vi "Detector Init.vi"(8 "error in (no error)":errorcluster, 10 "Detector Config":T2={"Detector"=0, "Offsets"=[[0, 0, 0, 0, 0, 0, 0, 0, 0, 0, 0, 0, 0, 0, 0, 0, 0, 0, 0, 0, 0, 0, 0, 0, 0, 0, 0, 0, 0, 0, 0, 0]], "Detector Computer"={"Machine"="192.168.121.11", "Password"="", "FITS File Path"="", "Port"=44444, "Header Path"="", "Name"=""}, "FITS hdr template0"=path "", "FITS hdr template1"=path "", "FITS Data File Path"=path "", "FITS Detector Settings"={"Exp Time Short"=0.0, "# of Frames"=0.0, "Exp Time Long"=0.0, "# of Groups"=0.0, "Object Name"="", "Object"="", "Obs Type"="", "Image Type"="", "Observer"="", "Observer Affiliation"=""}, "Sim Folder"=path "", "Integration Mode"=enum."Ramp", "Integration Time"=0.0, "Frame Int Time"=0.0} {"Offsets" format="%04x"; "Detector" items=["0", "1", "2"]}, 11 "PRIME Detector in":refnum<class "PRIME Detector.lvclass">) -> (0 "error out":errorcluster, 2 "Log Messages":string[](array[string]), 3 "PRIME Detector out":refnum<class "PRIME Detector.lvclass">)   [LabVIEW 2024, in "PRIME Detector.lvclass"]
uses:
  PRIME Detector.lvclass
  RIMAS Detector Config.ctl
  RIMAS Detector Server Config.ctl
  RIMAS Observation Config.ctl
  Detector enum Detector Integration Mode.ctl
  PRIME Detector cluster Status.ctl
  PRIME Detector.lvclass/PRIME Detector.ctl
  Detector Class.lvclass
panel:
  out "Status":T1
  # "sec"
  # "sec"
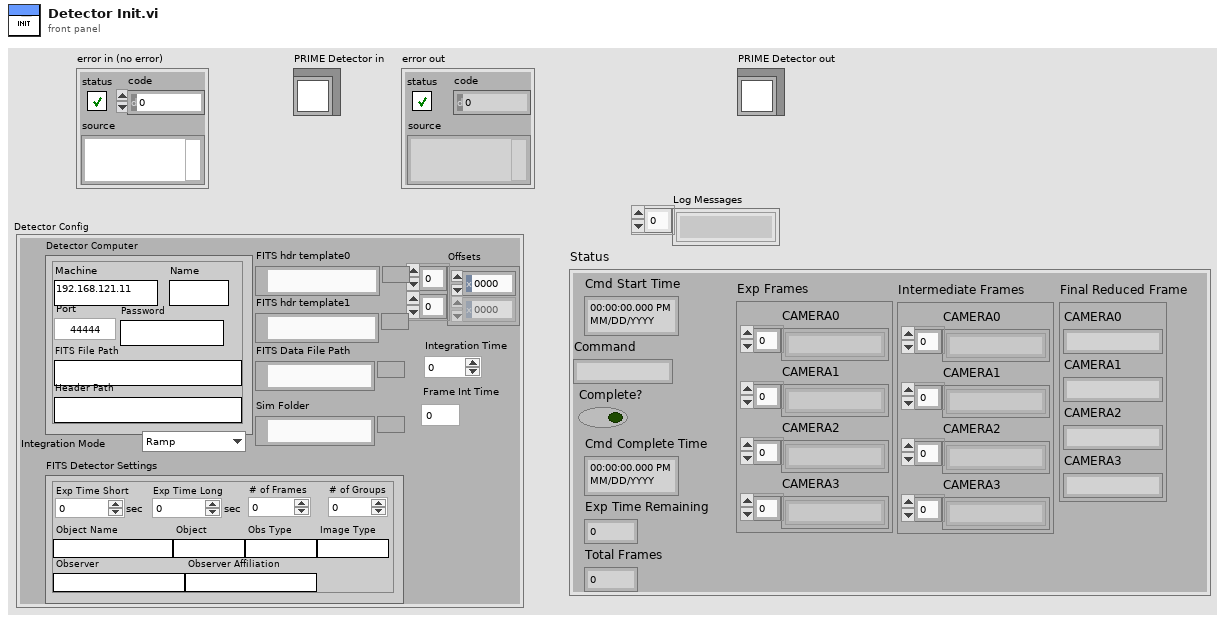
[diagram p1: front panel]
types:
  T1 = typedef "PRIME Detector cluster Status.ctl" = cluster{"Cmd Start Time":timestamp, "Command":string, "Complete?":bool, "Cmd Complete Time":timestamp, "Exp Time Remaining":dbl, "Total Frames":i32, "Exp Frames":cluster{"CAMERA0":string[], "CAMERA1":string[], "CAMERA2":string[], "CAMERA3":string[]}, "Intermediate Frames":cluster{"CAMERA0":string[], "CAMERA1":string[], "CAMERA2":string[], "CAMERA3":string[]}, "Final Reduced Frame":cluster{"CAMERA0":string, "CAMERA1":string, "CAMERA2":string, "CAMERA3":string}}
  T2 = typedef "RIMAS Detector Config.ctl" = cluster{"Detector":u16, "Offsets":u16[][], "Detector Computer":T3, "FITS hdr template0":path, "FITS hdr template1":path, "FITS Data File Path":path, "FITS Detector Settings":T4, "Sim Folder":path, "Integration Mode":T5, "Integration Time":dbl, "Frame Int Time":dbl}
  T3 = typedef "RIMAS Detector Server Config.ctl" = cluster{"Machine":string, "Password":string, "FITS File Path":string, "Port":u16, "Header Path":string, "Name":string}
  T4 = typedef "RIMAS Observation Config.ctl" = cluster{"Exp Time Short":dbl, "# of Frames":dbl, "Exp Time Long":dbl, "# of Groups":dbl, "Object Name":string, "Object":string, "Obs Type":string, "Image Type":string, "Observer":string, "Observer Affiliation":string}
  T5 = typedef "Detector enum Detector Integration Mode.ctl" = enum16{"Ramp", "CDS", "FOWLER2", "FOWLER4", "FOWLER8", "FOWLER16", "Raw"}
  T6 = typedef "PRIME Detector cluster Settings.ctl" = cluster{"Python Server":path}
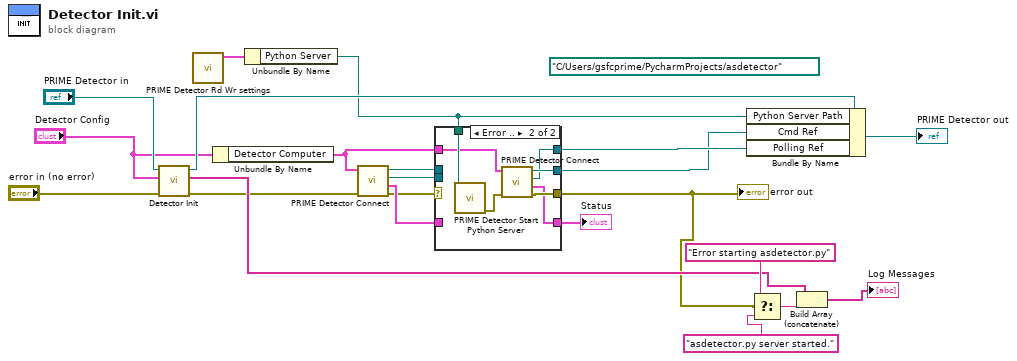
[diagram p0: block diagram]
diagram:
  (unwired) path "C:/Users/gsfcprime/PycharmProjects/asdetector" ("working directory")
  n1 = call-parent "Detector Init.vi"("error in (no error)"="error in (no error)", "Detector Config"="Detector Config", "Detector Class in"="PRIME Detector in") -> ("error out"=w11:errorcluster, "Log Messages"=w15:string[], "Detector Class out"=w20:refnum<class "PRIME Detector.lvclass">)  [unwired: 6 in]
  n2 = call "PRIME Detector Rd Wr settings.vi"() -> ("PRIME Detector Settings"=w12:T6)  [unwired: 10 in, 1 out]
  n3 = Unbundle By Name("Detector Config") -> ("Detector Computer"=w6:T3)
  n4 = Unbundle By Name(w12) -> ("Python Server"=w10:path)
  n5 = call "PRIME Detector Connect.vi"("error in (no error)"=w11, "Detector Computer"=w6) -> ("error out"=w3:errorcluster, "Status"=w4:T1, "Polling Ref"=w7:refnum<k5>, "Cmd Ref"=w9:refnum<k5>)  [unwired: 6 in]
  n6 = case shown="Error .." w3 {
    selector: w3 -> [w25 _]
    tunnel: w10 -> [_ w33]
    tunnel: w9 -> [w26 _]
    tunnel: [w26 w31] -> w1
    tunnel: [w25 w30] -> w2
    tunnel: [w23 w28] -> w8
    tunnel: w7 -> [w24 _]
    tunnel: w6 -> [_ w29]
    tunnel: [w24 w27] -> w5
    tunnel: w4 -> [w23 _]
    frame No Error {
    }
    frame Error {
      n7 = call "PRIME Detector Start Python Server.vi"("working directory"=w33) -> ("error out"=w32:errorcluster)  [unwired: 8 in, 2 out]
      n8 = call "PRIME Detector Connect.vi"("error in (no error)"=w32, "Detector Computer"=w29) -> ("error out"=w30:errorcluster, "Status"=w28:T1, "Polling Ref"=w27:refnum<k5>, "Cmd Ref"=w31:refnum<k5>)  [unwired: 6 in]
    }
  }
  "error out" <- w2
  "Status" <- w8
  n9 = Bundle By Name(cluster=w20, "Python Server Path"=w10, "Cmd Ref"=w1, "Polling Ref"=w5) -> (→"PRIME Detector out":refnum<class "PRIME Detector.lvclass">)
  n10 = Select(t="Error starting asdetector.py", s=w2, f="asdetector.py server started.") -> (s? t:f=w16:string)
  n11 = Build Array (concatenate)(w15, w16) -> (→"Log Messages":string[])
